vi "slope_to_rpm.vi"(9 "slope":dbl, 10 "Sampling Frequency [Hz]":dbl, 11 "Number of Stickers":i64) -> (3 "RPM":dbl)   [LabVIEW 2025, in "LabJackEKG.lvlib"]
uses:
  LabJackEKG.lvlib
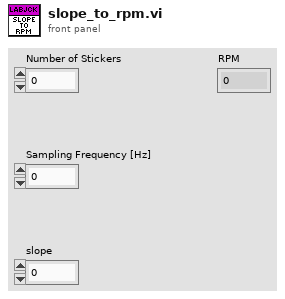
[diagram p1: front panel]
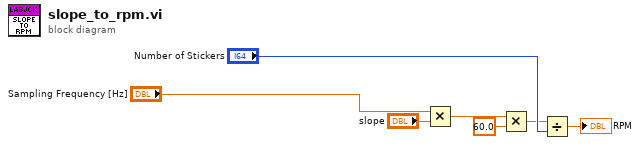
[diagram p0: block diagram]
diagram:
  n1 = Multiply(x="Sampling Frequency [Hz]", y="slope") -> (x*y=w2:dbl)
  n2 = Multiply(x=w2, y=60.0) -> (x*y=w1:dbl)
  n3 = Divide(x=w1, y="Number of Stickers") -> (x/y=→"RPM":dbl)
